vi "Run Sequence.vi"(0 "XNET Sesion":refnum<k21>, 1 "Console":refnum<vi>, 2 "Barcode":string, 11 "Error In":errorcluster) -> (4 "Pass":bool, 15 "Error Out":errorcluster)   [LabVIEW 2021]
doc: "Runs the actual IPC flash sequence. It will only pass if the DUT reports PCBAID 5 and Geneology reads back successfully."
uses:
  Controls/Sequence States.ctl
  <vilib>/xnet/xnet.llb/XNET Read (Signal Single-point).vi
  <vilib>/regexp/Match Regular Expression.xnode
panel:
  # "Inputs"
  # "Outputs"
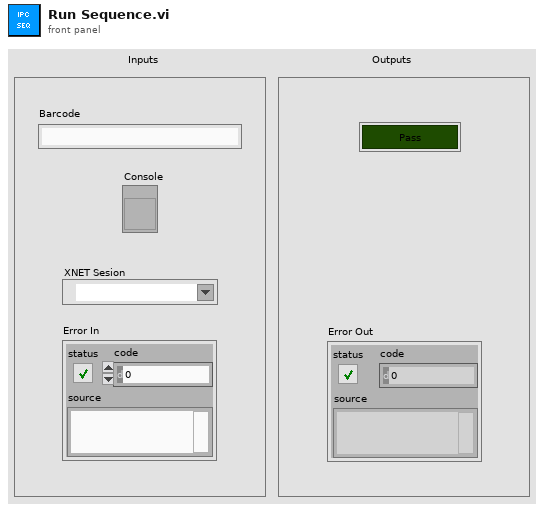
[diagram p1: front panel]
types:
  T1 = typedef "Sequence States.ctl" = enum16{"Check Barcode", "Check PCBAID", "Flash BL", "Confirm PCBAID", "Genealogy"}
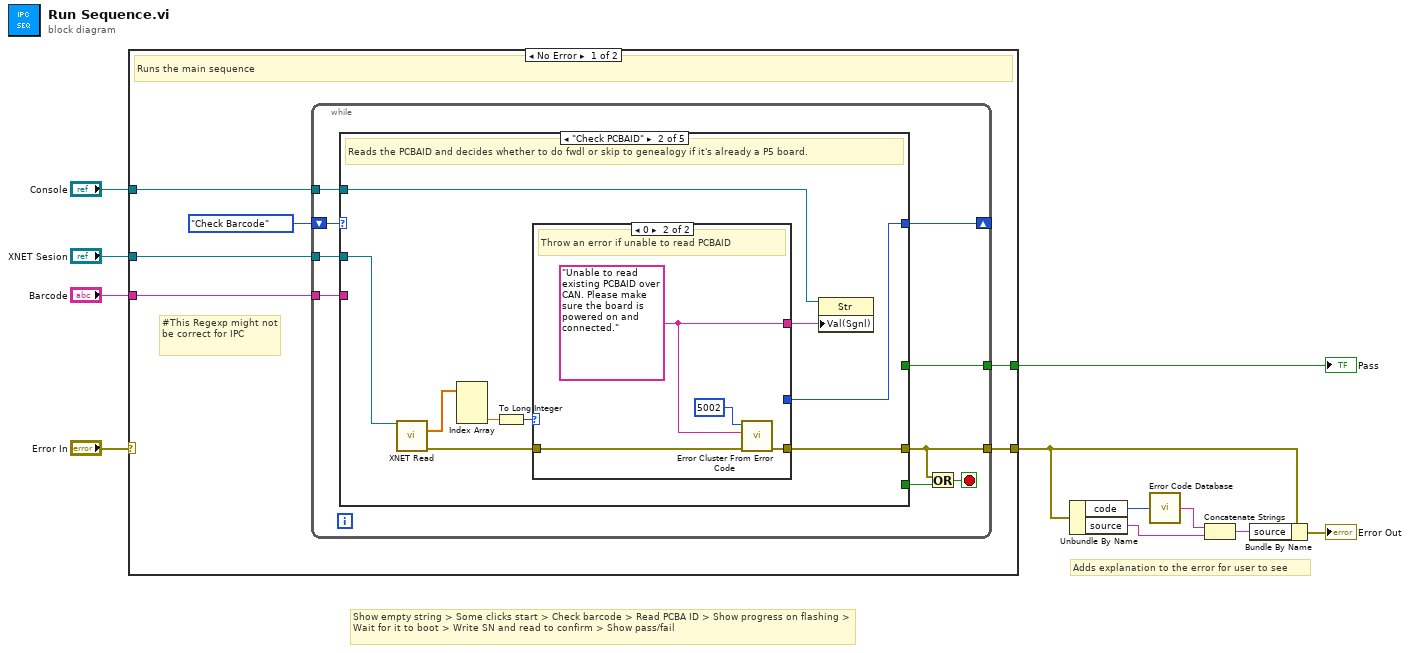
[diagram p0: block diagram]
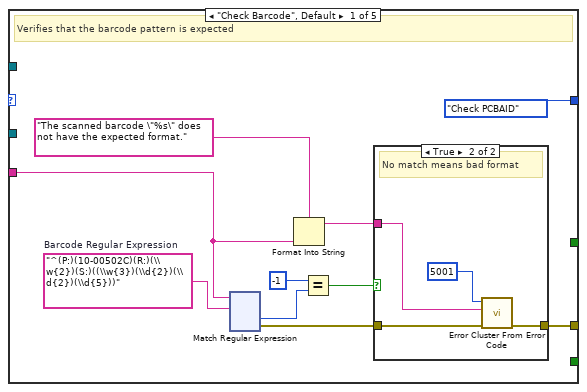
[diagram p2: hidden frame]
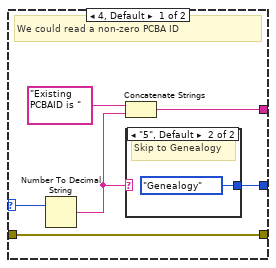
[diagram p4: hidden frame]
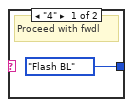
[diagram p5: hidden frame]
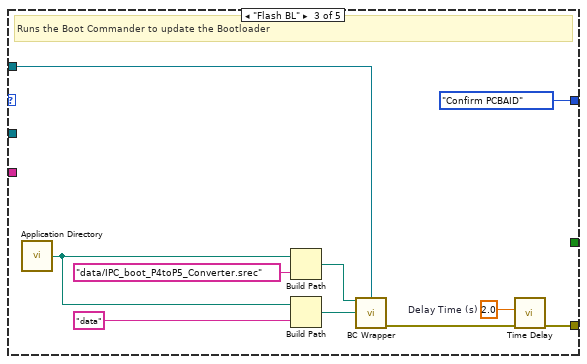
[diagram p6: hidden frame]
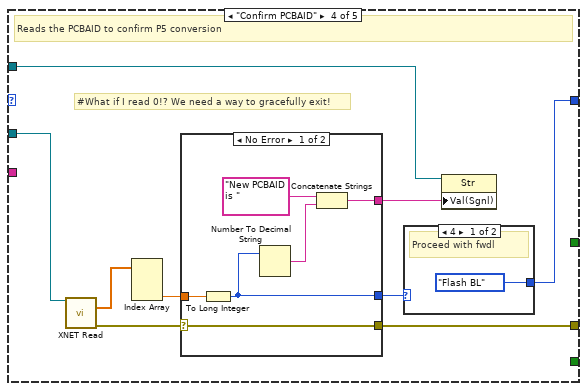
[diagram p7: hidden frame]
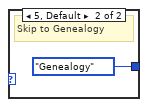
[diagram p8: hidden frame]
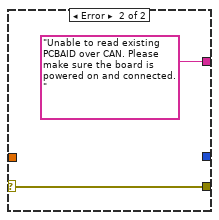
[diagram p9: hidden frame]
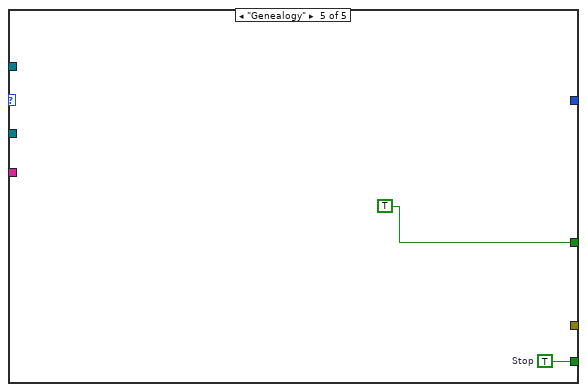
[diagram p10: hidden frame]
diagram:
  # "Adds explanation to the error for user to see"
  # "Show empty string > Some clicks start > Check barcode > Read PCBA ID > Show progress on flashing > Wait for it to boot > Write SN and read to confirm > Show pass/fail"
  n1 = case shown="No Error" "Error In" {
    selector: "Error In" -> [_ w211]
    tunnel: "Barcode" -> [w17 _]
    tunnel: [w16 w211] -> w5
    tunnel: "XNET Sesion" -> [w14 _]
    tunnel: "Console" -> [w13 _]
    tunnel: [w12 _] -> w1
    frame No Error {
      # "#This Regexp might not be correct for IPC"
      # "Runs the main sequence"
      n2 = while {
        shift-right: [w24] -> _
        shift-left: Sequence_States."Check Barcode" -> [w26]
        tunnel: w17 -> [w25]
        tunnel: [w20] -> w16
        tunnel: w14 -> [w23]
        tunnel: w13 -> [w22]
        tunnel: [w21] -> w12
        stop <- w19 stop-if-true
        n3 = case shown="\"Check PCBAID\"" w26 {
          tunnel: w25 -> [w27 _ _ _ _]
          tunnel: [w31 w160 w186 w195 _] -> w20
          tunnel: [Sequence_States."Check PCBAID" w159 Sequence_States."Confirm PCBAID" w190 _] -> w24
          tunnel: w23 -> [_ w167 _ w198 _]
          tunnel: w22 -> [_ w165 w188 w194 _]
          tunnel: [_ _ _ _ TRUE] -> w21
          tunnel: [_ _ _ _ w209] -> w18
          frame "Check Barcode", Default {
            w36 = "^(P:)(10-00502C)(R:)(\\w{2})(S:)((\\w{3})(\\d{2})(\\d{2})(\\d{5}))"  # Barcode Regular Expression
            # "Verifies that the barcode pattern is expected"
            n4 = xnode "Match Regular Expression"("input string"=w27, "regular expression"=w36) -> ("offset past match"=w35:i32, "error out"=w32:errorcluster)  [unwired: 4 in, 3 out]
            n5 = Format Into String(format string="The scanned barcode \"%s\" does not have the expected format.", w27) -> (resulting string=w28:string)  [unwired: 2 in, 1 out]
            n6 = Equal?(x=-1, y=w35) -> (x = y?=w30:bool)
            n7 = case shown="True" w30 {
              tunnel: w32 -> [w37 w41]
              tunnel: [w37 w40] -> w31
              tunnel: w28 -> [_ w38]
              frame False {
                # "Barcode format is OK"
              }
              frame True {
                # "No match means bad format"
                n8 = call <vilib>:"Error Cluster From Error Code.vi"("error in (no error)"=w41, "error message (\"\")"=w38, "error code (0)"=5001) -> ("error out"=w40:errorcluster)  [unwired: 6 in]
              }
            }
          }
          frame "Check PCBAID" {
            # "Reads the PCBAID and decides whether to do fwdl or skip to genealogy if it's already a P5 board."
            n9 = call-poly <vilib>:"XNET Read.vi"("session in"=w167) -> ("data"=w166:dbl[], "error out"=w161:errorcluster)  [unwired: 12 in, 1 out]
            n10 = Index Array(array=w166) -> (element #3=w163:dbl)  [unwired: 3 in, 2 out]
            n11 = To Long Integer(number=w163) -> (32bit integer=w162:i32)
            n12 = case shown="0" w162 {
              selector: w162 -> [w171 _]
              tunnel: [w172 w176] -> w164
              tunnel: w161 -> [w170 w179]
              tunnel: [w170 w178] -> w160
              tunnel: [w168 _] -> w159
              frame 4, Default {
                # "We could read a non-zero PCBA ID"
                n13 = Number To Decimal String(number=w171) -> (decimal integer string=w169:string)  [unwired: 1 in]
                n14 = Concatenate Strings("Existing PCBAID is ", w169) -> (w172:string)
                n15 = case shown="\"5\", Default" w169 {
                  tunnel: [Sequence_States."Flash BL" Sequence_States."Genealogy"] -> w168
                  frame "4" {
                    # "Proceed with fwdl"
                  }
                  frame "5", Default {
                    # "Skip to Genealogy"
                  }
                }
              }
              frame 0 {
                w176 = "Unable to read existing PCBAID over CAN. Please make sure the board is powered on and connected."
                # "Throw an error if unable to read PCBAID"
                n16 = call <vilib>:"Error Cluster From Error Code.vi"("error in (no error)"=w179, "error message (\"\")"=w176, "error code (0)"=5002) -> ("error out"=w178:errorcluster)  [unwired: 6 in]
              }
            }
            n17 = property class="Str"(reference=w165, "Val(Sgnl)"=w164) -> ()  [unwired: 1 in, 2 out]
          }
          frame "Flash BL" {
            w185 = 2.0  # Delay Time (s)
            # "Runs the Boot Commander to update the Bootloader"
            n18 = call <vilib>:"Application Directory.vi"() -> ("Application Directory"=w182:path)
            n19 = Build Path(base path=w182, name or relative path="data/IPC_boot_P4toP5_Converter.srec") -> (appended path=w183:path)
            n20 = Build Path(base path=w182, name or relative path="data") -> (appended path=w184:path)
            n21 = call "BC Wrapper.vi"("File To Program"=w183, "Console Ref"=w188, "BootCommander Folder"=w184) -> ("error out"=w187:errorcluster)  [unwired: 10 in, 2 out]
            n22 = call "Time Delay"("error in (no error)"=w187, "Delay Time (s)"=w185) -> ("error out"=w186:errorcluster)  [unwired: 9 in]
          }
          frame "Confirm PCBAID" {
            # "#What if I read 0!? We need a way to gracefully exit!"
            # "Reads the PCBAID to confirm P5 conversion"
            n23 = call-poly <vilib>:"XNET Read.vi"("session in"=w198) -> ("data"=w197:dbl[], "error out"=w196:errorcluster)  [unwired: 12 in, 1 out]
            n24 = Index Array(array=w197) -> (element #3=w192:dbl)  [unwired: 3 in, 2 out]
            n25 = case shown="No Error" w196 {
              selector: w196 -> [w202 w208]
              tunnel: [w202 w208] -> w195
              tunnel: [w204 "Unable to read existing PCBAID over CAN. Please make sure the board is powered on and connected."] -> w193
              tunnel: w192 -> [w205 _]
              tunnel: [w201 _] -> w191
              frame No Error {
                n26 = To Long Integer(number=w205) -> (32bit integer=w201:i32)
                n27 = Number To Decimal String(number=w201) -> (decimal integer string=w203:string)  [unwired: 1 in]
                n28 = Concatenate Strings("New PCBAID is ", w203) -> (w204:string)
              }
              frame Error {
              }
            }
            n29 = case shown="4" w191 {
              tunnel: [Sequence_States."Flash BL" Sequence_States."Genealogy"] -> w190
              frame 4 {
                # "Proceed with fwdl"
              }
              frame 5, Default {
                # "Skip to Genealogy"
              }
            }
            n30 = property class="Str"(reference=w194, "Val(Sgnl)"=w193) -> ()  [unwired: 1 in, 2 out]
          }
          frame "Genealogy" {
            w209 = TRUE  # Stop
          }
        }
        n31 = Or(x=w20, y=w18) -> (x .or. y?=w19:bool)
      }
    }
    frame Error {
      # "Can't start due to error"
    }
  }
  "Pass" <- w1
  n32 = Unbundle By Name(w5) -> ("code"=w9:i32, "source"=w8:string)
  n33 = call <vilib>:"Error Code Database.vi"("Error Code"=w9) -> ("Error Text"=w7:string)
  n34 = Concatenate Strings(w7, w8) -> (w6:string)
  n35 = Bundle By Name(cluster=w5, "source"=w6) -> (→"Error Out":errorcluster)
